vi "Get Freq-RPM Spectral Map.vi"   [LabVIEW 2017, in "SoundVib_Gabor.lvlib"]
doc: "Generates a frequency-rpm spectral map of the data block referenced by <B>RefNum in</B>. You can use this polymorphic VI to return <B>spectral map</B> as a 2D array of double-precision, floating-point numbers or a 2D array of 8-bit unsigned integers. You must manually select the polymorphic instance to use. Use the DBL instance to obtain more accurate data. Use the U8 instance to reduce memory usage when the VI displays data."
uses:
  <vilib>/addons/Sound and Vibration/Order Analysis/Gabor Order Tracking/SoundVib_Gabor.lvlib
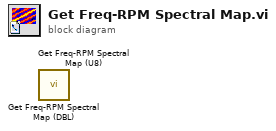
[diagram p0: block diagram]
diagram:
  n1 = call <vilib>:"Get Freq-RPM Spectral Map (DBL).vi"() -> ()  [unwired: 6 in, 6 out]
  n2 = call <vilib>:"Get Freq-RPM Spectral Map (U8).vi"() -> ()  [unwired: 6 in, 6 out]
